vi "TIFF-Create IFD.vi"(0 "height":u32, 5 "width":u32, 7 "max frames":u16=1, 9 "Image size (bytes)":u32, 11 "error in":errorcluster, 12 "byte order":T1(ring)=enum."little-endian") -> (4 "unsigned byte array":u8[](array[numeric]), 15 "error out":errorcluster)   [LabVIEW 2020]
doc: "This VI writes an image array to a multipage tif file. Valid formats are U8 or U16."
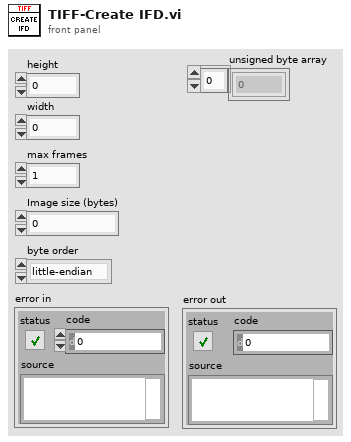
[diagram p1: front panel]
types:
  T1 = enum16{"big-endian, network order", "native, host order", "little-endian"}
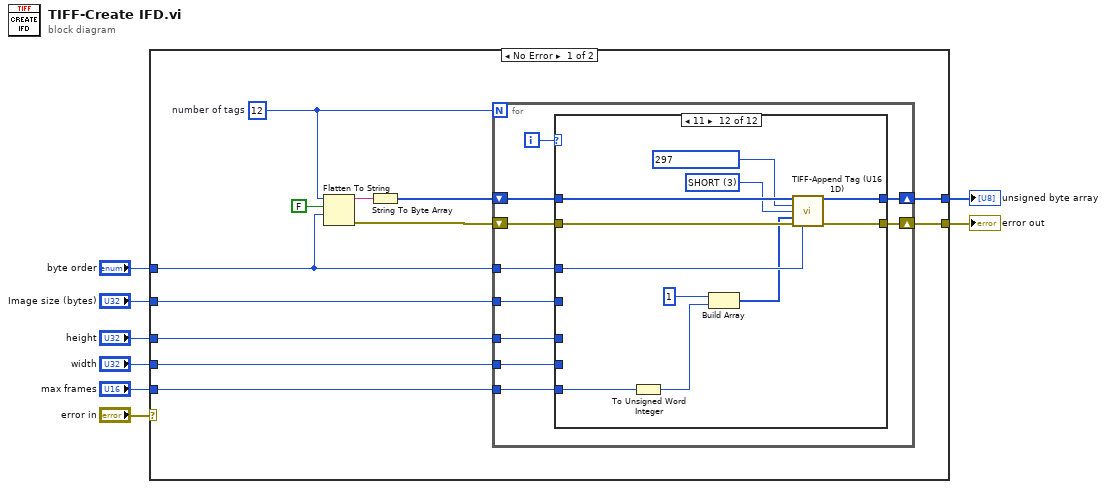
[diagram p0: block diagram]
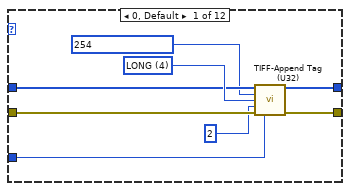
[diagram p2: hidden frame]
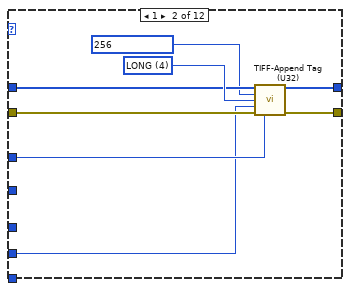
[diagram p3: hidden frame]
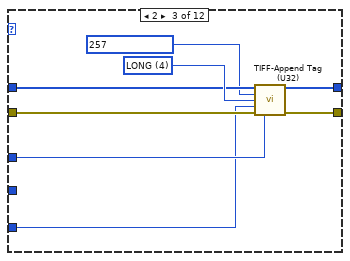
[diagram p4: hidden frame]
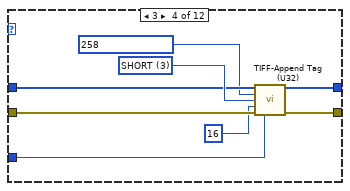
[diagram p5: hidden frame]
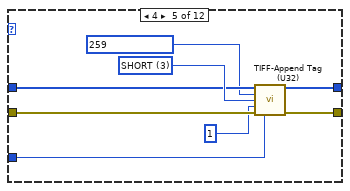
[diagram p6: hidden frame]
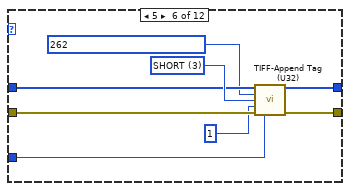
[diagram p7: hidden frame]
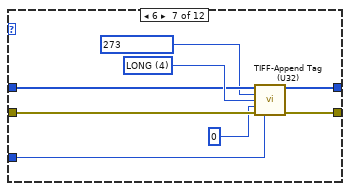
[diagram p8: hidden frame]
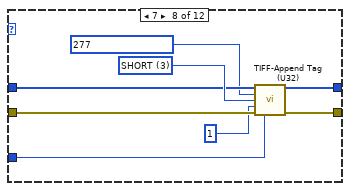
[diagram p9: hidden frame]
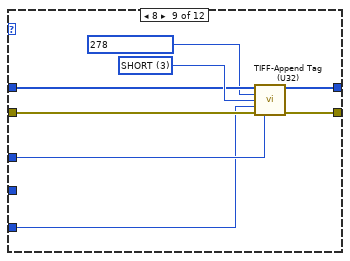
[diagram p10: hidden frame]
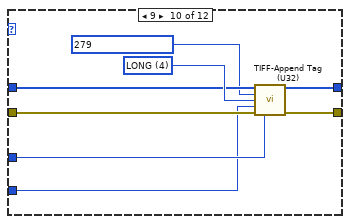
[diagram p11: hidden frame]
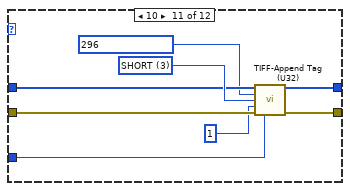
[diagram p12: hidden frame]
diagram:
  n1 = case shown="No Error" "error in" {
    selector: "error in" -> [_ w130]
    tunnel: "height" -> [w20 _]
    tunnel: "width" -> [w19 _]
    tunnel: "byte order" -> [w18 _]
    tunnel: [w17 _] -> w5
    tunnel: [w11 w130] -> w3
    tunnel: "max frames" -> [w10 _]
    tunnel: "Image size (bytes)" -> [w9 _]
    frame No Error {
      w14 = u16 12  # number of tags
      n2 = Flatten To String(anything=w14, prepend array or string size? (T)=FALSE, byte order (0:big-endian, network order)=w18) -> (data string=w16:string, error out=w12:errorcluster)  [unwired: 1 in, 1 out]
      n3 = String To Byte Array(string=w16) -> (unsigned byte array=w13:u8[])
      n4 = for {
        N: w14 -> [_]
        tunnel: w20 -> [w30]
        tunnel: w19 -> [w29]
        tunnel: w18 -> [w28]
        shift-right: [w24] -> w17
        shift-left: w13 -> [w26]
        shift-right: [w23] -> w11
        shift-left: w12 -> [w25]
        tunnel: w10 -> [w22]
        tunnel: w9 -> [w21]
        i -> [w27]
        n5 = case shown="11" w27 {
          tunnel: w30 -> [_ _ w47 _ _ _ _ _ w95 _ _ _]
          tunnel: w29 -> [_ w39 _ _ _ _ _ _ _ _ _ _]
          tunnel: w28 -> [w34 w42 w50 w58 w66 w74 w82 w90 w98 w106 w114 w123]
          tunnel: w26 -> [w33 w41 w49 w57 w65 w73 w81 w89 w97 w105 w113 w126]
          tunnel: w25 -> [w38 w46 w54 w62 w70 w78 w86 w94 w102 w110 w118 w128]
          tunnel: [w36 w44 w52 w60 w68 w76 w84 w92 w100 w108 w116 w129] -> w24
          tunnel: [w35 w43 w51 w59 w67 w75 w83 w91 w99 w107 w115 w127] -> w23
          tunnel: w22 -> [_ _ _ _ _ _ _ _ _ _ _ w119]
          tunnel: w21 -> [_ _ _ _ _ _ _ _ _ w103 _ _]
          frame 0, Default {
            w37 = u16 4 items=["BYTE"=1, "ASCII"=2, "SHORT"=3, "LONG"=4, "RATIONAL"=5] ("DataType")
            n6 = call "TIFF-Append Tag (U32).vi"("IFD in"=w33, "[IN] TagID"=u16 254 ("BaselineTags"), "[IN] DataType"=w37, "[IN] Data"=u32 2, "error IN"=w38, "[IN] Byte order"=w34) -> ("IFD out"=w36:u8[], "error OUT"=w35:errorcluster)  [unwired: 8 in]
          }
          frame 1 {
            w45 = u16 4 items=["BYTE"=1, "ASCII"=2, "SHORT"=3, "LONG"=4, "RATIONAL"=5] ("DataType")
            n7 = call "TIFF-Append Tag (U32).vi"("IFD in"=w41, "[IN] TagID"=u16 256 ("BaselineTags"), "[IN] DataType"=w45, "[IN] Data"=w39, "error IN"=w46, "[IN] Byte order"=w42) -> ("IFD out"=w44:u8[], "error OUT"=w43:errorcluster)  [unwired: 8 in]
          }
          frame 2 {
            w53 = u16 4 items=["BYTE"=1, "ASCII"=2, "SHORT"=3, "LONG"=4, "RATIONAL"=5] ("DataType")
            n8 = call "TIFF-Append Tag (U32).vi"("IFD in"=w49, "[IN] TagID"=u16 257 ("BaselineTags"), "[IN] DataType"=w53, "[IN] Data"=w47, "error IN"=w54, "[IN] Byte order"=w50) -> ("IFD out"=w52:u8[], "error OUT"=w51:errorcluster)  [unwired: 8 in]
          }
          frame 3 {
            w61 = u16 3 items=["BYTE"=1, "ASCII"=2, "SHORT"=3, "LONG"=4, "RATIONAL"=5] ("DataType")
            n9 = call "TIFF-Append Tag (U32).vi"("IFD in"=w57, "[IN] TagID"=u16 258 ("BaselineTags"), "[IN] DataType"=w61, "[IN] Data"=u32 16, "error IN"=w62, "[IN] Byte order"=w58) -> ("IFD out"=w60:u8[], "error OUT"=w59:errorcluster)  [unwired: 8 in]
          }
          frame 4 {
            w69 = u16 3 items=["BYTE"=1, "ASCII"=2, "SHORT"=3, "LONG"=4, "RATIONAL"=5] ("DataType")
            n10 = call "TIFF-Append Tag (U32).vi"("IFD in"=w65, "[IN] TagID"=u16 259 ("BaselineTags"), "[IN] DataType"=w69, "[IN] Data"=u32 1, "error IN"=w70, "[IN] Byte order"=w66) -> ("IFD out"=w68:u8[], "error OUT"=w67:errorcluster)  [unwired: 8 in]
          }
          frame 5 {
            w77 = u16 3 items=["BYTE"=1, "ASCII"=2, "SHORT"=3, "LONG"=4, "RATIONAL"=5] ("DataType")
            n11 = call "TIFF-Append Tag (U32).vi"("IFD in"=w73, "[IN] TagID"=u16 262 ("BaselineTags"), "[IN] DataType"=w77, "[IN] Data"=u32 1, "error IN"=w78, "[IN] Byte order"=w74) -> ("IFD out"=w76:u8[], "error OUT"=w75:errorcluster)  [unwired: 8 in]
          }
          frame 6 {
            w85 = u16 4 items=["BYTE"=1, "ASCII"=2, "SHORT"=3, "LONG"=4, "RATIONAL"=5] ("DataType")
            n12 = call "TIFF-Append Tag (U32).vi"("IFD in"=w81, "[IN] TagID"=u16 273 ("BaselineTags"), "[IN] DataType"=w85, "[IN] Data"=u32 0, "error IN"=w86, "[IN] Byte order"=w82) -> ("IFD out"=w84:u8[], "error OUT"=w83:errorcluster)  [unwired: 8 in]
          }
          frame 7 {
            w93 = u16 3 items=["BYTE"=1, "ASCII"=2, "SHORT"=3, "LONG"=4, "RATIONAL"=5] ("DataType")
            n13 = call "TIFF-Append Tag (U32).vi"("IFD in"=w89, "[IN] TagID"=u16 277 ("BaselineTags"), "[IN] DataType"=w93, "[IN] Data"=u32 1, "error IN"=w94, "[IN] Byte order"=w90) -> ("IFD out"=w92:u8[], "error OUT"=w91:errorcluster)  [unwired: 8 in]
          }
          frame 8 {
            w101 = u16 3 items=["BYTE"=1, "ASCII"=2, "SHORT"=3, "LONG"=4, "RATIONAL"=5] ("DataType")
            n14 = call "TIFF-Append Tag (U32).vi"("IFD in"=w97, "[IN] TagID"=u16 278 ("BaselineTags"), "[IN] DataType"=w101, "[IN] Data"=w95, "error IN"=w102, "[IN] Byte order"=w98) -> ("IFD out"=w100:u8[], "error OUT"=w99:errorcluster)  [unwired: 8 in]
          }
          frame 9 {
            w109 = u16 4 items=["BYTE"=1, "ASCII"=2, "SHORT"=3, "LONG"=4, "RATIONAL"=5] ("DataType")
            n15 = call "TIFF-Append Tag (U32).vi"("IFD in"=w105, "[IN] TagID"=u16 279 ("BaselineTags"), "[IN] DataType"=w109, "[IN] Data"=w103, "error IN"=w110, "[IN] Byte order"=w106) -> ("IFD out"=w108:u8[], "error OUT"=w107:errorcluster)  [unwired: 8 in]
          }
          frame 10 {
            w117 = u16 3 items=["BYTE"=1, "ASCII"=2, "SHORT"=3, "LONG"=4, "RATIONAL"=5] ("DataType")
            n16 = call "TIFF-Append Tag (U32).vi"("IFD in"=w113, "[IN] TagID"=u16 296 ("BaselineTags"), "[IN] DataType"=w117, "[IN] Data"=u32 1, "error IN"=w118, "[IN] Byte order"=w114) -> ("IFD out"=w116:u8[], "error OUT"=w115:errorcluster)  [unwired: 8 in]
          }
          frame 11 {
            w124 = u16 3 items=["BYTE"=1, "ASCII"=2, "SHORT"=3, "LONG"=4, "RATIONAL"=5] ("DataType")
            n17 = To Unsigned Word Integer(number=w119) -> (unsigned 16bit integer=w121:u16)
            n18 = Build Array(u16 1 ("number"), w121) -> (w120:u16[])
            n19 = call "TIFF-Append Tag (U16 1D).vi"("IFD in"=w126, "[IN] TagID"=u16 297 ("BaselineTags"), "[IN] DataType"=w124, "[IN] Data"=w120, "error IN"=w128, "[IN] Byte order"=w123) -> ("IFD out"=w129:u8[], "error OUT"=w127:errorcluster)  [unwired: 8 in]
          }
        }
      }
    }
    frame Error {
    }
  }
  "error out" <- w3
  "unsigned byte array" <- w5
